vi "Read Instrument Name.vi"(8 "error in (no error)":errorcluster, 11 "Dynamic Instrument in":refnum<class "Dynamic Instrument.lvclass">) -> (0 "error out":errorcluster, 2 "Instrument Name":string, 3 "Dynamic Instrument out":refnum<class "Dynamic Instrument.lvclass">)   [LabVIEW 2016, in "Dynamic Instrument.lvlib" / "Dynamic Instrument.lvclass"]
uses:
  Dynamic Instrument.lvclass
  Dynamic Instrument.lvclass/Dynamic Instrument.ctl
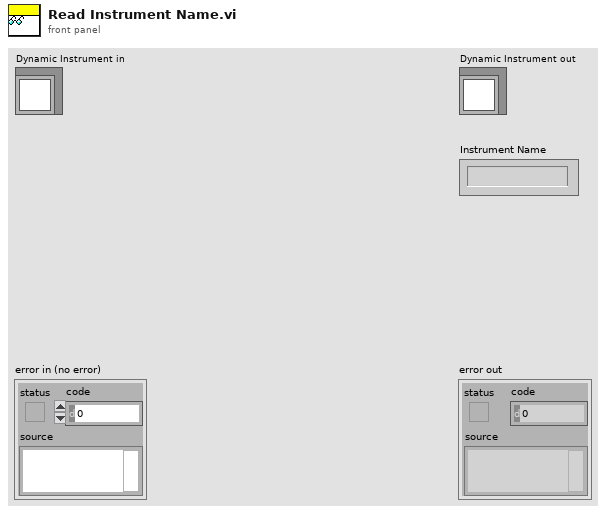
[diagram p1: front panel]
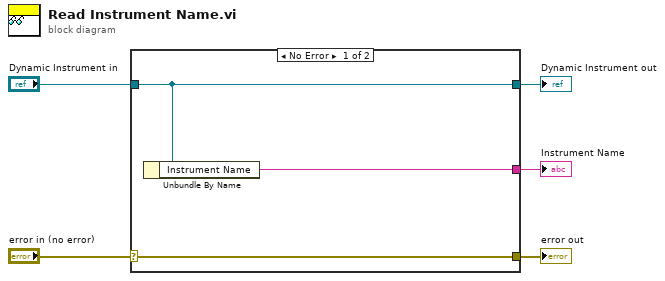
[diagram p0: block diagram]
diagram:
  n1 = case shown="No Error" "error in (no error)" {
    selector: "error in (no error)" -> [w8 w9]
    tunnel: [w8 w9] -> w4
    tunnel: [w7 w10] -> w2
    tunnel: "Dynamic Instrument in" -> [w7 w10]
    tunnel: [w6 _] -> w1
    frame No Error {
      n2 = Unbundle By Name(w7) -> ("Instrument Name"=w6:string)
    }
    frame Error {
    }
  }
  "error out" <- w4
  "Dynamic Instrument out" <- w2
  "Instrument Name" <- w1
